vi "hidSPD Read Report.vi"(8 "error in (no error)":errorcluster, 10 "timeout":i32=100, 11 "deviceInfo in":string) -> (0 "error out":errorcluster, 2 "hidSPD Simple Report":T1, 3 "deviceInfo out":string)   [LabVIEW 2018, in "hidSPDLibForLabView.lvlib"]
uses:
  hidSPDLibForLabView.lvlib
  hidSPD Controls/hidSPD Simple Report.ctl
  <vilib>/Utility/error.llb/Error Cluster From Error Code.vi
  <vilib>/ErrorRing/Error Ring.xnode
  hidSPD DLL files/libSPD.dll
panel:
  out "id":i32 format="%02x"
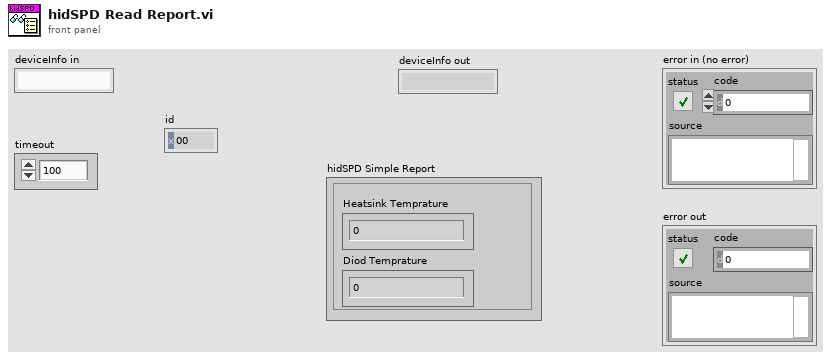
[diagram p1: front panel]
types:
  T1 = typedef "hidSPDLibForLabView.lvlib/hidSPD Simple Report.ctl" = cluster{"Heatsink Temprature":sgl, "Diod Temprature":sgl, "TEC-voltage":sgl, "Diod Bias":sgl, "RF Power":sgl, "Thermal used":sgl, "hv bias used":sgl, "hv code used":u16, "strobe code used":u16, "SPD number":u16, "SPD ready":u16}
  T2 = enum16{"big-endian, network order", "native, host order", "little-endian"}
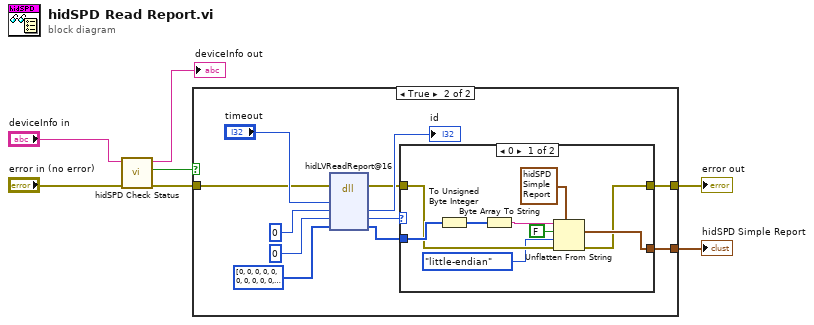
[diagram p0: block diagram]
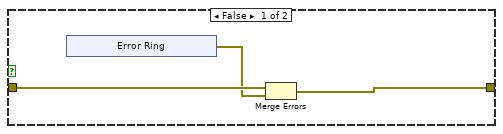
[diagram p2: hidden frame]
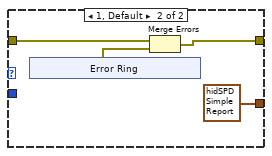
[diagram p3: hidden frame]
diagram:
  n1 = call "hidSPD Check Status.vi"("error in (no error)"="error in (no error)", "deviceInfo in"="deviceInfo in") -> ("error out"=w3:errorcluster, "available"=w4:bool, "deviceInfo out"=→"deviceInfo out":string)  [unwired: 7 in]
  n2 = case shown="True" w4 {
    tunnel: w3 -> [w10 w18]
    tunnel: [w8 w17] -> w2
    tunnel: [_ w16] -> w1
    frame False {
      n3 = xnode "Error Ring"() -> ("error out"=w9:errorcluster)
      n4 = Merge Errors(w10, w9) -> (w8:errorcluster)
    }
    frame True {
      n5 = dll-call lib="F:/NextCloud/SPD stand/hidSPDLibForLabView/hidSPD DLL files/libSPD.dll" fn="hidLVReadReport@16"(error in=w18, "timeout"="timeout", "id"=0 ("report"), "cmd"=0, "data"=i32[] [0, 0, 0, 0, 0, 0, 0, 0, 0, 0, 0, 0, 0, 0, 0, 0, 0, 0, 0, 0, 0, 0, 0, 0, 0, 0, 0, 0, 0, 0, 0, 0, 0, 0, 0, 0, 0, 0, 0, 0, 0, 0, 0, 0, 0, 0, 0, 0, 0, 0, 0, 0, 0, 0, 0, 0, 0, 0, 0, 0, 0, 0]) -> (error out=w20:errorcluster, "id"=→"id":i32, "cmd"=w21:i32, "data"=w22:i32[])  [unwired: 4 in, 1 out]
      n6 = case shown="0" w21 {
        tunnel: w22 -> [w35 _]
        tunnel: w20 -> [w31 w39]
        tunnel: [w29 w37] -> w17
        tunnel: [w30 T1 {"Heatsink Temprature"=0.0, "Diod Temprature"=0.0, "TEC-voltage"=0.0, "Diod Bias"=0.0, "RF Power"=0.0, "Thermal used"=0.0, "hv bias used"=0.0, "hv code used"=0, "strobe code used"=0, "SPD number"=0, "SPD ready"=0} ("hidSPD Simple Report")] -> w16
        frame 0 {
          n7 = To Unsigned Byte Integer(number=w35) -> (unsigned 8bit integer=w34:u8[])
          n8 = Byte Array To String(unsigned byte array=w34) -> (string=w33:string)
          n9 = Unflatten From String(type=T1 {"Heatsink Temprature"=0.0, "Diod Temprature"=0.0, "TEC-voltage"=0.0, "Diod Bias"=0.0, "RF Power"=0.0, "Thermal used"=0.0, "hv bias used"=0.0, "hv code used"=0, "strobe code used"=0, "SPD number"=0, "SPD ready"=0} ("hidSPD Simple Report"), binary string=w33, data includes array or string size? (T)=FALSE, byte order (0:big-endian, network order)=T2."little-endian", error in (no error)=w31) -> (value=w30:T1, error out=w29:errorcluster)  [unwired: 1 out]
        }
        frame 1, Default {
          n10 = xnode "Error Ring"() -> ("error out"=w38:errorcluster)
          n11 = Merge Errors(w39, w38) -> (w37:errorcluster)
        }
      }
    }
  }
  "error out" <- w2
  "hidSPD Simple Report" <- w1
